vi "Alarma_blink_control.vi"(1 "Nombre":string="Generador2", 2 "alarm":bool) -> ()   [LabVIEW 2018]
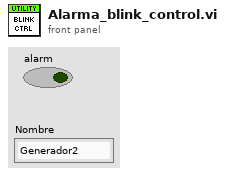
[diagram p1: front panel]
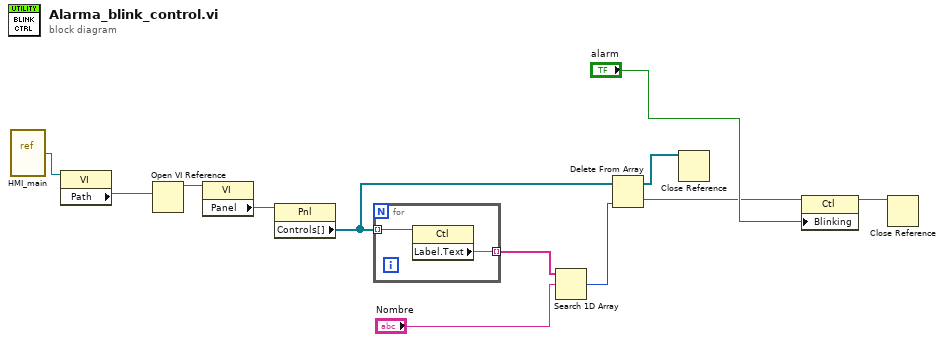
[diagram p0: block diagram]
diagram:
  n1 = vi-ref "HMI_main.vi"() -> (w2:refnum<vi>)
  n2 = property class="VI"(reference=w2) -> ("Path"=w1:path)  [unwired: 1 in, 2 out]
  n3 = Open VI Reference(vi path=w1) -> (vi reference=w4:refnum<vi>)  [unwired: 5 in, 1 out]
  n4 = property class="VI"(reference=w4) -> ("Panel"=w3:refnum<vi>)  [unwired: 1 in, 2 out]
  n5 = property class="Pnl"(reference=w3) -> ("Controls[]"=w7:refnum<vi>[])  [unwired: 1 in, 2 out]
  n6 = for {
    tunnel: w7 -> [w14] mode=indexing
    tunnel: [w13] -> w5 mode=indexing
    n7 = property class="Ctl"(reference=w14) -> ("Label.Text"=w13:string)  [unwired: 1 in, 2 out]
  }
  n8 = Search 1D Array(1D array=w5, element="Nombre") -> (index of element=w8:i32)  [unwired: 1 in]
  n9 = Delete From Array(array=w7, index=w8) -> (deleted portion=w10:refnum<vi>, array with subset deleted=w9:refnum<vi>[])  [unwired: 1 in]
  n10 = Close Reference(reference=w9) -> ()  [unwired: 1 in, 1 out]
  n11 = property class="Ctl"(reference=w10, "Blinking"="alarm") -> (reference out=w11:refnum<vi>)  [unwired: 1 in, 1 out]
  n12 = Close Reference(reference=w11) -> ()  [unwired: 1 in, 1 out]
